vi "myRIO_BRig_FPGA_stateSelection__v3.vi"(0 "I_selectionState":bool, 2 "I_selectRight":bool, 3 "I_selectWrong":bool, 5 "I_Left(F)_or_Right(T)":bool, 6 "I_ignoreWrong":bool, 8 "I_lickL":bool, 10 "I_lickR":bool, 14 "I_allReward":bool) -> (22 "output__I_selectRight":bool, 23 "output__I_selectWrong":bool)   [LabVIEW 2014]
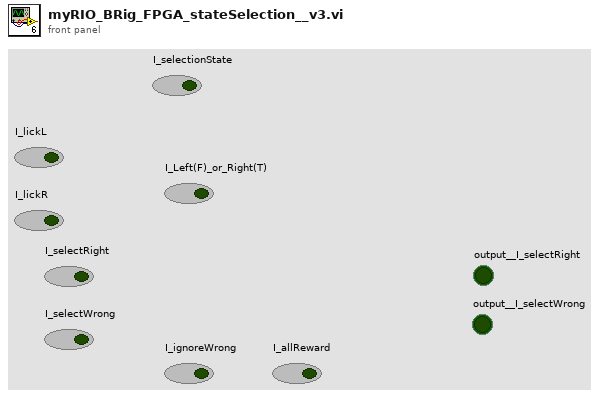
[diagram p1: front panel]
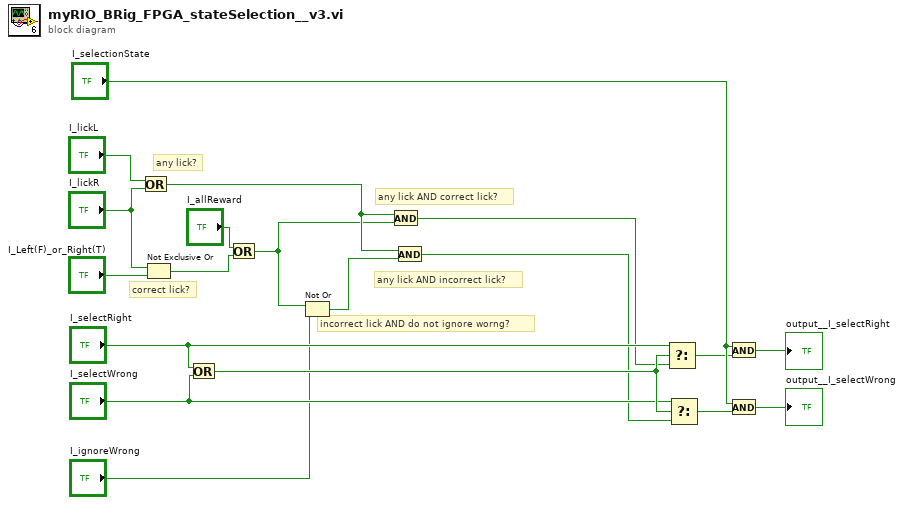
[diagram p0: block diagram]
diagram:
  # "incorrect lick AND do not ignore worng?"
  # "any lick AND incorrect lick?"
  # "any lick AND correct lick?"
  # "any lick?"
  # "correct lick?"
  n1 = Or(x="I_lickL", y="I_lickR") -> (x .or. y?=w5:bool)
  n2 = Not Exclusive Or(1:"I_Left(F)_or_Right(T)", 2:"I_lickR") -> (0:w3:bool)
  n3 = Or(x="I_selectRight", y="I_selectWrong") -> (x .or. y?=w12:bool)
  n4 = Or(x="I_allReward", y=w3) -> (x .or. y?=w1:bool)
  n5 = Not Or(1:"I_ignoreWrong", 2:w1) -> (0:w7:bool)
  n6 = And(x=w5, y=w1) -> (x .and. y?=w4:bool)
  n7 = And(x=w5, y=w7) -> (x .and. y?=w6:bool)
  n8 = Select(t="I_selectRight", s=w12, f=w4) -> (s? t:f=w9:bool)
  n9 = Select(t="I_selectWrong", s=w12, f=w6) -> (s? t:f=w13:bool)
  n10 = And(x="I_selectionState", y=w9) -> (x .and. y?=→"output__I_selectRight":bool)
  n11 = And(x="I_selectionState", y=w13) -> (x .and. y?=→"output__I_selectWrong":bool)
